vi "Test Map Range Overflow to Multiple Ranges.vi"(8 "error in (no error)":errorcluster, 11 "Test Case In":refnum<class "Revisit Test.lvclass">) -> (0 "error out":errorcluster, 3 "Test Case Out":refnum<class "Revisit Test.lvclass">)   [LabVIEW 2020, in "Revisit Test.lvclass"]
uses:
  Revisit Test.lvclass
  C:/Program Files (x86)/National Instruments/LabVIEW 2020/vi.lib/Astemes/LUnit/Test Case.lvclass
  <vilib>/Astemes/LUnit/Test Case.lvclass/Test Case.ctl
  4993e8ee-a06a-463a-9684-69129f64d5ce.vi
  <vilib>/Astemes/LUnit/Append Pass Result.vi
  <vilib>/Astemes/LUnit/Append Fail Result.vi
  <vilib>/Astemes/LUnit/Describe Comparison.vi
  <vilib>/Astemes/LUnit/Compare Variants.vi
  <vilib>/Astemes/LUnit/Variant to string.vi
  <vilib>/Utility/Data Type/Get Type Information.vi
  <vilib>/Utility/LVClass/Get LV Class Name.vi
  Range Map/Range Map.lvclass
  Range/Range.lvclass
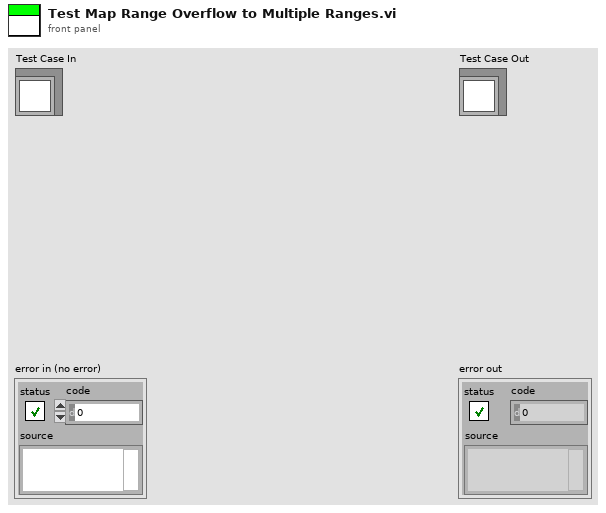
[diagram p1: front panel]
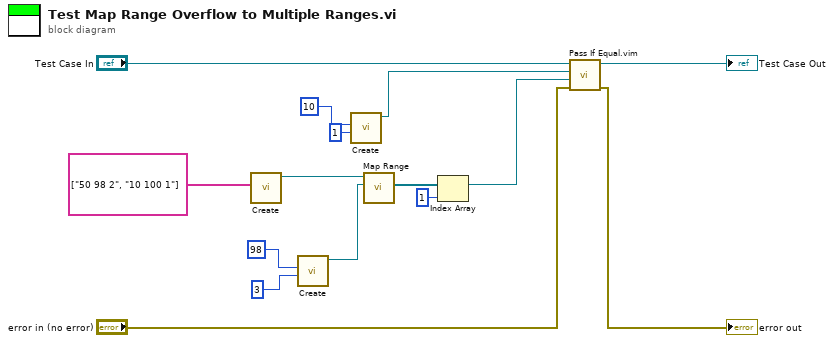
[diagram p0: block diagram]
diagram:
  n1 = call "Create.vi"("Input"=string[] ["50 98 2", "10 100 1"] ("string array")) -> ("Range Map"=w9:refnum<class "Range Map.lvclass">)  [unwired: 9 in, 1 out]
  n2 = call "Create.vi"("Length"=u64 3, "From"=u64 98) -> ("Range"=w8:refnum<class "Range.lvclass">)  [unwired: 8 in, 1 out]
  n3 = call "Create.vi"("Length"=u64 1, "From"=u64 10) -> ("Range"=w6:refnum<class "Range.lvclass">)  [unwired: 8 in, 1 out]
  n4 = call "Map Range.vi"("Range"=w8, "Range Map in"=w9) -> ("Ranges"=w5:refnum<class "Range.lvclass">[])  [unwired: 7 in, 2 out]
  n5 = Index Array(array=w5, index=1) -> (element=w2:refnum<class "Range.lvclass">)
  n6 = call "Pass If Equal.vim"("error in (no error)"="error in (no error)", "Actual"=w2, "Expected"=w6, "LUnit Test Case In"="Test Case In") -> ("error out"=→"error out":errorcluster, "LUnit Test Case Out"=→"Test Case Out":refnum<class "Revisit Test.lvclass">)  [unwired: 6 in]
